vi "Run.vi"(8 "error in (no error)":errorcluster caption="entrée d'erreur (pas d'erreur)", 11 "Kddcup99.lvclass":refnum<class "Kddcup99.lvclass">) -> (0 "error in (no error)":errorcluster caption="entrée d'erreur (pas d'erreur)", 2 "Data":T1, 3 "Kddcup99.lvclass":refnum<class "Kddcup99.lvclass">)   [LabVIEW 2020, in "Kddcup99.lvclass"]
doc: "Returns :\n\n- data : ndarray of shape (494021, 41)\nThe data matrix to learn.\n\n- target : ndarray of shape (494021,)\nThe regression target for each sample."
uses:
  Kddcup99.lvclass
  Kddcup99.lvclass/Kddcup99.ctl
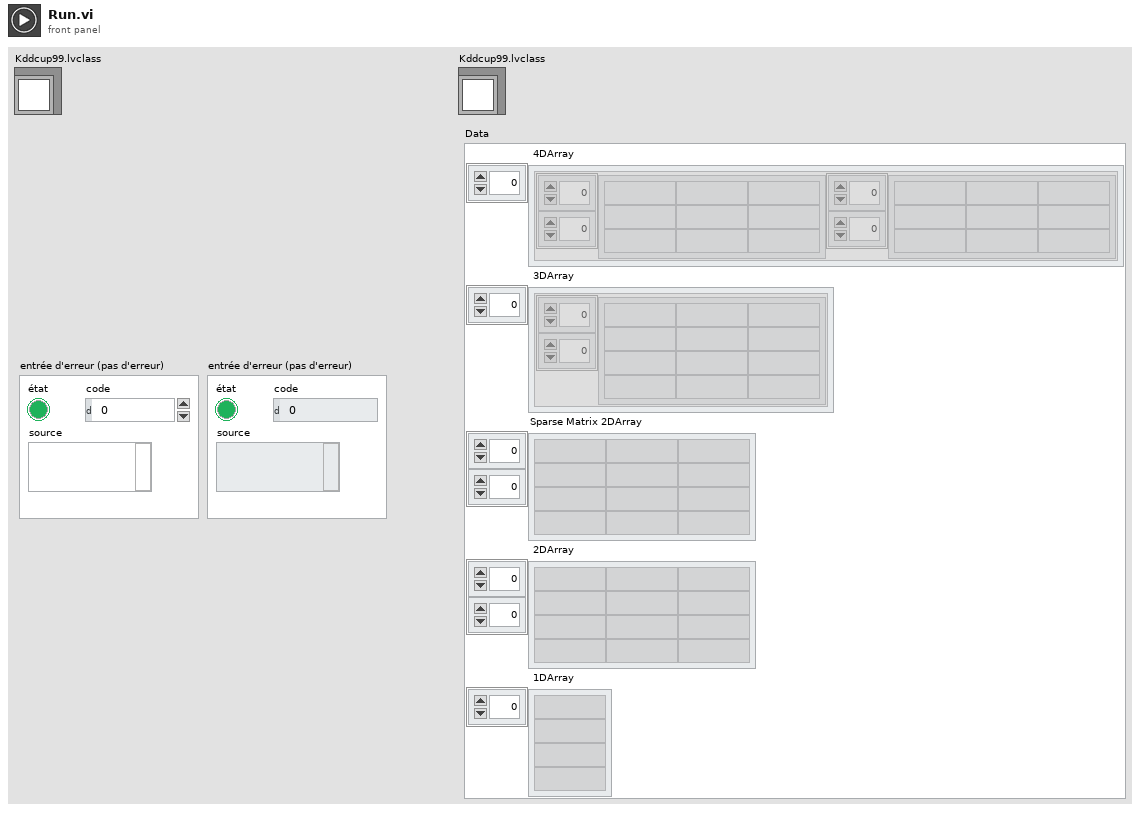
[diagram p1: front panel]
types:
  T1 = cluster{" 4DArray":cluster{"1":string[][], "2":string[][]}[], " 3DArray":cluster{"Tableau":string[][]}[], "Sparse Matrix 2DArray":string[][], " 2DArray":string[][], " 1DArray":string[]}
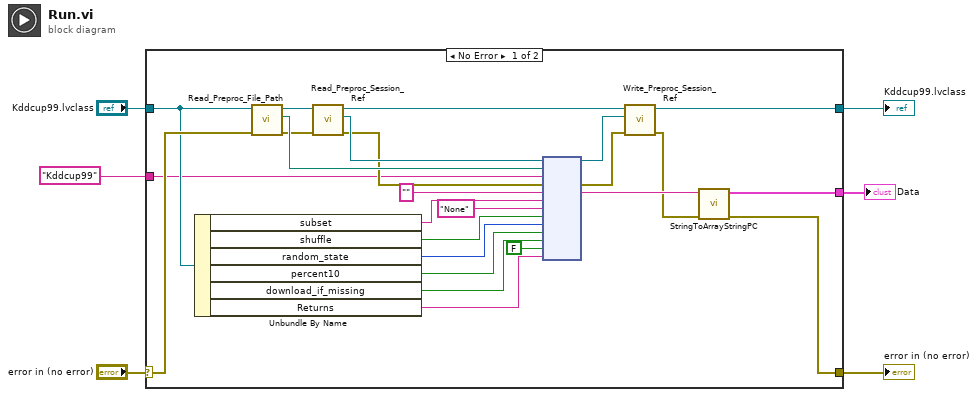
[diagram p0: block diagram]
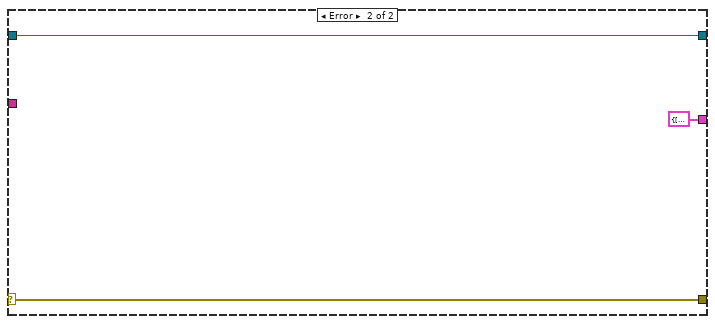
[diagram p2: hidden frame]
diagram:
  n1 = case shown="No Error" "error in (no error)" {
    selector: "error in (no error)" -> [w22 w34]
    tunnel: [w8 w34] -> w5
    tunnel: [w11 w33] -> w3
    tunnel: "Kddcup99.lvclass" -> [w21 w33]
    tunnel: "Kddcup99" -> [w20 _]
    tunnel: [w7 T1 {" 4DArray"=[], " 3DArray"=[], "Sparse Matrix 2DArray"=[], " 2DArray"=[], " 1DArray"=[]} ("Data")] -> w1
    frame No Error {
      n2 = Unbundle By Name(w21) -> ("subset"=w19:string, "shuffle"=w17:bool, "random_state"=w16:i32, "percent10"=w15:bool, "download_if_missing"=w14:bool, "Returns"=w12:string)
      n3 = call-dynamic "Read_Preproc_File_Path.vi"("error in (no error)"=w22, "Python in"=w21) -> ("error out"=w26:errorcluster, "File_Path"=w29:path, "Python out"=w31:refnum<class "Kddcup99.lvclass">)  [unwired: 7 in]
      n4 = call-dynamic "Read_Preproc_Session_Ref.vi"("error in (no error)"=w26, "Python in"=w31) -> ("error out"=w27:errorcluster, "Session_ref"=w28:refnum<k35>, "Python out"=w30:refnum<class "Kddcup99.lvclass">)  [unwired: 7 in]
      n5 = node(w28, w29, w20, w27, "", w19, "None", w17, w16, w15, w14, FALSE, w12) -> (w23:refnum<k35>, w25:errorcluster, w10:string)  [unwired: 8 in, 2 out]
      n6 = call-dynamic "Write_Preproc_Session_Ref.vi"("error in (no error)"=w25, "Session_ref"=w23, "Python in"=w30) -> ("error out"=w9:errorcluster, "Python out"=w11:refnum<class "Kddcup99.lvclass">)  [unwired: 7 in]
      n7 = call "StringToArrayStringPC.vi"("sortie d'erreur"=w9, "Return value"=w10) -> ("sortie d'erreur"=w8:errorcluster, "Data"=w7:T1)  [unwired: 8 in]
    }
    frame Error {
    }
  }
  "error in (no error)" <- w5
  "Kddcup99.lvclass" <- w3
  "Data" <- w1
